vi "Get Object Item (single) by Path.vi"(7 "Item Path":string, 8 "error in (no error)":errorcluster, 10 "Object Offset":i32, 11 "JSON":string) -> (0 "error out":errorcluster, 1 "<JSON>":string caption="JSON substring", 2 "Item offset":i32, 3 "Found":bool)   [LabVIEW 2013, in "JSONtext.lvlib"]
uses:
  JSONtext.lvlib
  support/JSONtext support.lvlib
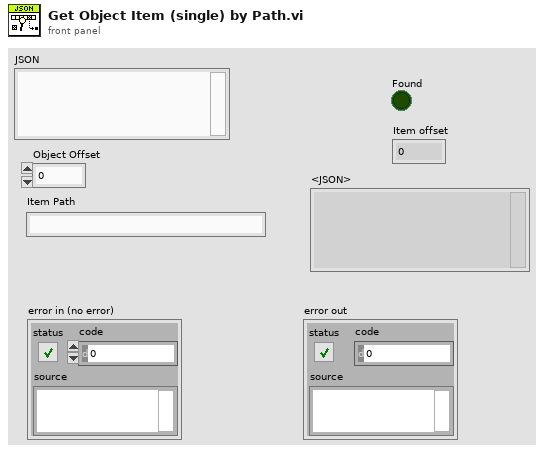
[diagram p1: front panel]
types:
  T1 = typedef "JSONtext.lvlib/Found Items.ctl" = cluster{"Item offset":i32, "Offset past Item":i32, "Name offset":i32, "Offset past Name":i32, "Found":bool, "Empty Object":bool}
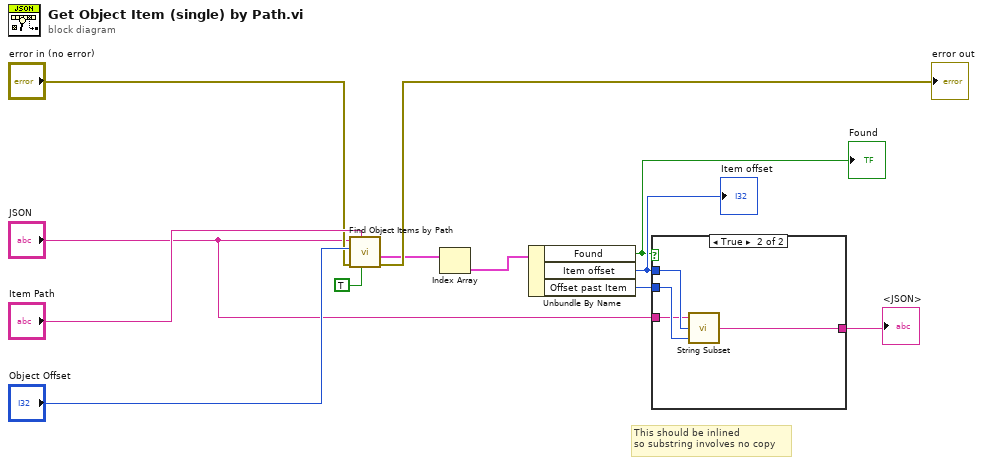
[diagram p0: block diagram]
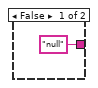
[diagram p2: hidden frame]
diagram:
  # "This should be inlined\nso substring involves no copy"
  n1 = call "Find Object Items by Path.vi"("Only return first found"=TRUE, "Path"="Item Path", "error in (no error)"="error in (no error)", "Object Offset"="Object Offset", "JSON"="JSON") -> ("error out"=→"error out":errorcluster, "Items"=w6:T1[])  [unwired: 5 in]
  n2 = Index Array(array=w6) -> (element=w5:T1)  [unwired: 1 in]
  n3 = Unbundle By Name(w5) -> ("Found"=w2:bool, "Item offset"=w4:i32, "Offset past Item"=w3:i32)
  "Found" <- w2
  "Item offset" <- w4
  n4 = case shown="True" w2 {
    tunnel: "JSON" -> [_ w14]
    tunnel: ["null" ("substring") w17] -> w1
    tunnel: w4 -> [_ w16]
    tunnel: w3 -> [_ w15]
    frame False {
    }
    frame True {
      n5 = call "String Subset.vi"("Offset past End"=w15, "Start offset"=w16, "JSON"=w14) -> ("substring"=w17:string)  [unwired: 2 in]
    }
  }
  "<JSON>" <- w1
